vi "SetVerboseMode.vi"(8 "error in (no error)":errorcluster, 10 "Verbosity":enum16{"Off", "On"}(ring), 11 "ControlState in":T1 {"ChainMask" format="0x%02x"}) -> (0 "error out":errorcluster, 3 "ControlState out":T1 {"ChainMask" format="0x%02x"})   [LabVIEW 2023, in "ArduinoSerialBling.lvlib"]
uses:
  ArduinoSerialBling.lvlib
  ControlState.ctl
  ChainState.ctl
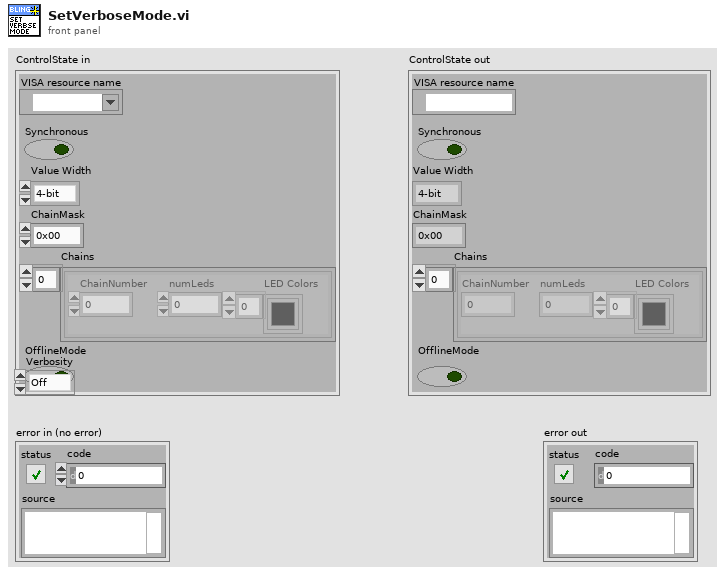
[diagram p1: front panel]
types:
  T1 = typedef "ArduinoSerialBling.lvlib/ControlState.ctl" = cluster{"VISA resource name":refnum<visa-resource-name>, "Synchronous":bool, "Value Width":enum16{"4-bit", "8-bit"}, "ChainMask":u8, "Chains":T2[], "OfflineMode":bool}
  T2 = typedef "ArduinoSerialBling.lvlib/ChainState.ctl" = cluster{"ChainNumber":u8, "numLeds":u8, "LED Colors":u32[]}
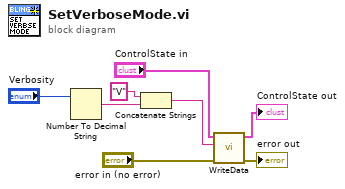
[diagram p0: block diagram]
diagram:
  n1 = Number To Decimal String(number="Verbosity") -> (decimal integer string=w6:string)  [unwired: 1 in]
  n2 = Concatenate Strings("V" ("write buffer"), w6) -> (w2:string)
  n3 = call "WriteData.vi"("error in (no error)"="error in (no error)", "Command"=w2, "ControlState in"="ControlState in") -> ("error out"=→"error out":errorcluster, "ControlState out"=→"ControlState out":T1)  [unwired: 5 in, 2 out]
